vi "Set Ramp.vi"(8 "error in (no error)":errorcluster, 9 "Output #":i32=1, 10 "Ramp rate (0: off)":dbl, 11 "Cryo-Con Driver in":refnum<class "Cryo-Con Driver.lvclass">) -> (0 "error out":errorcluster, 3 "Cryo-Con Driver out":refnum<class "Cryo-Con Driver.lvclass">)   [LabVIEW 2021, in "Cryo-Con Driver.lvclass"]
uses:
  Cryo-Con Driver.lvclass
  C:/GitHub/NHMFL_Core/Libraries/Instruments/VISA Instrument/VISA Instrument.lvclass
  C:/GitHub/NHMFL_Core/Libraries/Instruments/Temperature Controller Driver/Temperature Controller Driver.lvclass
  VISA Instrument/VISA Instrument.lvclass/VISA Instrument.ctl
  VISA Instrument/Read VISA resource.vi
  VISA Instrument/Write VISA resource.vi
  Temperature Controller Driver/Read T controller configuration.vi
  Cryo-Con Driver.lvclass/Cryo-Con Driver.ctl
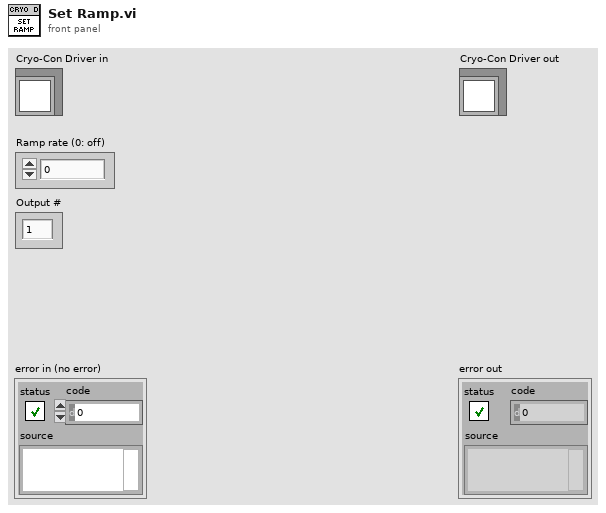
[diagram p1: front panel]
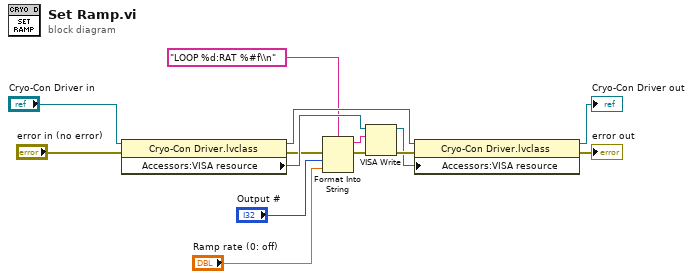
[diagram p0: block diagram]
diagram:
  n1 = property class="Cryo-Con Driver.lvclass"(reference="Cryo-Con Driver in", error in="error in (no error)") -> (reference out=w14:refnum<class "Cryo-Con Driver.lvclass">, error out=w8:errorcluster, "Accessors:VISA resource"=w9:refnum<visa-resource-name>)
  n2 = Format Into String(format string="LOOP %d:RAT %#f\\n", error in=w8, "Output #", "Ramp rate (0: off)") -> (resulting string=w3:string, error out=w4:errorcluster)  [unwired: 1 in]
  n3 = VISA Write(VISA resource name=w9, write buffer=w3, error in (no error)=w4) -> (VISA resource name out=w6:refnum<visa-resource-name>, error out=w7:errorcluster)  [unwired: 1 out]
  n4 = property class="Cryo-Con Driver.lvclass"(reference=w14, error in=w7, "Accessors:VISA resource"=w6) -> (reference out=→"Cryo-Con Driver out":refnum<class "Cryo-Con Driver.lvclass">, error out=→"error out":errorcluster)
